vi "外观判断DB.vi"(1 "点数":i32, 4 "起点":i32) -> (0 "结果":string)   [LabVIEW 2018]
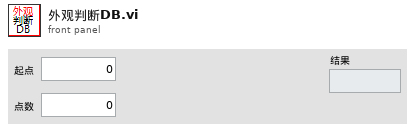
[diagram p1: front panel]
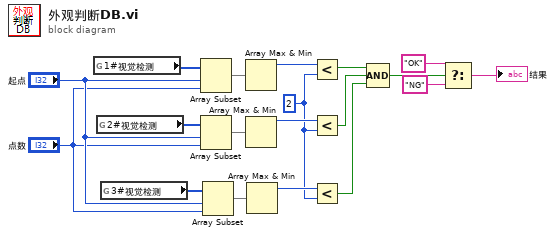
[diagram p0: block diagram]
diagram:
  w8 = u16 2
  n1 = global read "全局 1.vi" "1#视觉检测"() -> (w19:u16[])
  n2 = global read "全局 1.vi" "2#视觉检测"() -> (w18:u16[])
  n3 = global read "全局 1.vi" "3#视觉检测"() -> (w15:u16[])
  n4 = Array Subset(array=w19, index="起点", length="点数") -> (w14:u16[])
  n5 = Array Subset(array=w18, index="起点", length="点数") -> (w13:u16[])
  n6 = Array Subset(array=w15, index="起点", length="点数") -> (w12:u16[])
  n7 = Array Max & Min(array=w14) -> (max value=w11:u16)  [unwired: 3 out]
  n8 = Array Max & Min(array=w13) -> (max value=w10:u16)  [unwired: 3 out]
  n9 = Array Max & Min(array=w12) -> (max value=w9:u16)  [unwired: 3 out]
  n10 = Less?(x=w11, y=w8) -> (x < y?=w7:bool)
  n11 = Less?(x=w10, y=w8) -> (x < y?=w6:bool)
  n12 = Less?(x=w9, y=w8) -> (x < y?=w5:bool)
  n13 = Compound Arithmetic op=AND ("复合运算")(w7, w6, w5) -> (w4:bool)
  n14 = Select(t="OK", s=w4, f="NG") -> (s? t:f=→"结果":string)
